vi "PI-Double To String.vi"(2 "Start":dbl, 3 "String in":string) -> (0 "String out":string)   [LabVIEW 2020]
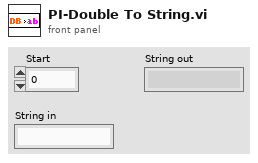
[diagram p1: front panel]
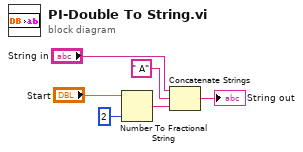
[diagram p0: block diagram]
diagram:
  n1 = Number To Fractional String(number="Start", precision (6)=i16 2) -> (F-format string=w2:string)  [unwired: 2 in]
  n2 = Concatenate Strings("String in", " A", w2) -> (→"String out":string)
